vi "GLdrv_Open_USB.vi"(0 "ID":i32) -> (4 "Connection ID":T1, 15 "error out":errorcluster)   [LabVIEW 2017]
uses:
  ConnectionID.ctl
  gtcusbr.dll
  GL860_Driver.lvlib
panel:
  in  "TCP/IP dmy":refnum<k5>
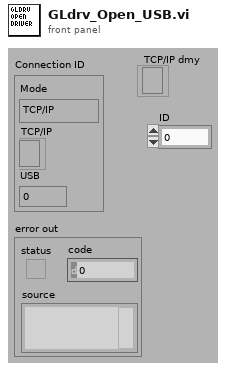
[diagram p1: front panel]
types:
  T1 = typedef "ConnectionID.ctl" = cluster{"Mode":enum16{"TCP/IP", "USB"}, "TCP/IP":refnum<k5>, "USB":i32}
  T2 = cluster{"Mode":enum16{"TCP/IP", "USB"}, "TCP/IP dmy":refnum<k5>, "HANDLE":i32}
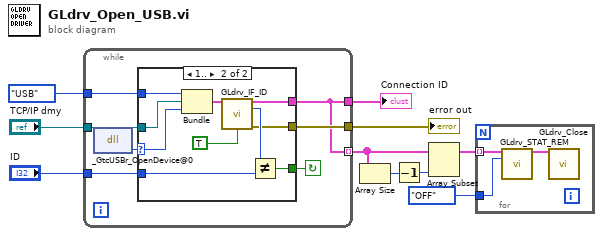
[diagram p0: block diagram]
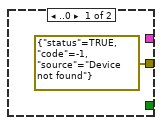
[diagram p2: hidden frame]
diagram:
  n1 = while {
    tunnel: enum16{"TCP/IP", "USB"}."USB" ("Mode") -> [w17]
    tunnel: "TCP/IP dmy" -> [w16]
    tunnel: [w11] -> w8
    tunnel: [w14] -> w7
    tunnel: "ID" -> [w12]
    tunnel: [w11] -> w5 mode=indexing
    stop <- w13 continue-if-true
    n2 = dll-call lib="D:/src/LabVIEW/GL860/JP/LabView VI/Driver/gtcusbr.dll" fn="_GtcUSBr_OpenDevice@0"() -> ("HANDLE"=w15:i32)  [unwired: 3 in, 2 out]
    n3 = case shown="1.." w15 {
      selector: w15 -> [_ w26]
      tunnel: w17 -> [_ w28]
      tunnel: w16 -> [_ w27]
      tunnel: [_ w22] -> w11
      tunnel: [errorcluster {"status"=TRUE, "code"=-1, "source"="Device not found"} ("error out") w19] -> w14
      tunnel: [_ w24] -> w13
      tunnel: w12 -> [_ w25]
      frame ..0 {
      }
      frame 1.. {
        n4 = Bundle("Mode"=w28, "TCP/IP dmy"=w27, "HANDLE"=w26) -> (w23:T2)  [unwired: 1 out]
        n5 = call "GLdrv_IF_ID.vi"("Connection ID"=w23, "Query(f)"=TRUE) -> ("Connection ID Out"=w22:T1, "ID out"=w21:i32, "error out"=w19:errorcluster)  [unwired: 2 in, 9 out]
        n6 = Not Equal?(x=w21, y=w25) -> (x != y?=w24:bool)
      }
    }
  }
  "Connection ID" <- w8
  "error out" <- w7
  n7 = Array Size(array=w5) -> (size(s)=w3:i32)
  n8 = Decrement(x=w3) -> (x-1=w2:i32)
  n9 = Array Subset(array=w5, length=w2) -> (w4:T1[])  [unwired: 1 in]
  n10 = for {
    tunnel: w4 -> [w31] mode=indexing
    tunnel: enum16{"ON", "OFF"}."OFF" ("Remote") -> [w29]
    n11 = call "GLdrv_STAT_REM.vi"("Connection ID"=w31, "Remote"=w29) -> ("Connection ID Out"=w30:T1)  [unwired: 1 in, 12 out]
    n12 = call "GLdrv_Close.vi"("Connection ID Out"=w30) -> ()  [unwired: 1 in, 14 out]
  }
